vi "get aggregate names.vi"() -> (2 "section names":string[](array[string]), 3 "Refnum out":T1)   [LabVIEW 2019]
uses:
  <vilib>/Utility/config.llb/Config Data RefNum.ctl
  <vilib>/Utility/sysdir.llb/System Directory Type.ctl
  <vilib>/Utility/config.llb/NI_LVConfig.lvlib
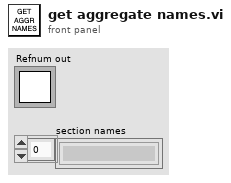
[diagram p1: front panel]
types:
  T1 = typedef "NI_LVConfig.lvlib/Config Data RefNum.ctl" = refnum<k1>
  T2 = typedef "System Directory Type.ctl" = i32
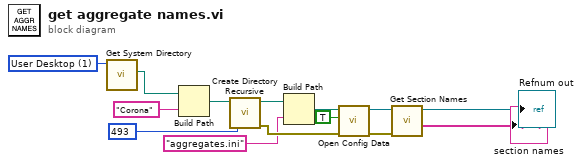
[diagram p0: block diagram]
diagram:
  w1 = T2 1 items=["User Home"=0, "User Desktop"=1, "User Documents"=2, "User Application Data"=3, "User Preferences"=4, "User Temporary"=5, "Public Documents"=6, "Public Application Data"=7, "Public Preferences"=8, "Public Cache"=13, "System Core Libraries"=9, "System Installed Libraries"=10, "Application Files"=11, "Boot Volume Root"=12] ("system directory type")
  n1 = call <vilib>:"Get System Directory.vi"("system directory type"=w1) -> ("system directory"=w2:path)  [unwired: 10 in]
  n2 = Build Path(base path=w2, name or relative path="Corona") -> (appended path=w9:path)
  n3 = call <vilib>:"Create Directory Recursive.vi"("permissions"=i16 493, "directory"=w9) -> ("error out"=w11:errorcluster, "directory copy"=w10:path)  [unwired: 3 in, 1 out]
  n4 = Build Path(base path=w10, name or relative path="aggregates.ini") -> (appended path=w5:path)
  n5 = call <vilib>:"Open Config Data.vi"("error in (no error)"=w11, "create file if necessary (T)"=TRUE, "configuration file path"=w5) -> ("error out"=w8:errorcluster, "refnum"=w7:T1)  [unwired: 6 in, 1 out]
  n6 = call <vilib>:"Get Section Names.vi"("error in (no error)"=w8, "refnum"=w7) -> ("section names"=→"section names":string[], "refnum out"=→"Refnum out":T1)  [unwired: 7 in, 1 out]
